vi "GEN_Time-coded_overlay_PIC.vi"(7 "Image size":cluster{"x":i32, "y":i32}={"x"=480, "y"=480}, 8 "Error In":errorcluster, 9 "Samples full merge, every N":i32=10000, 10 "Multiline grouping, samples":i32=100, 11 "Full track array":T1(array[cluster])) -> (0 "Error Out":errorcluster, 3 "Time-coded overlay pixmap":u32[][](array[numeric]) format="%x")   [LabVIEW 2018, in "Tracker.lvlib"]
uses:
  Tracker.lvlib
  Controls/CTL_Color_ramp.ctl
  Common_Resources.lvlib
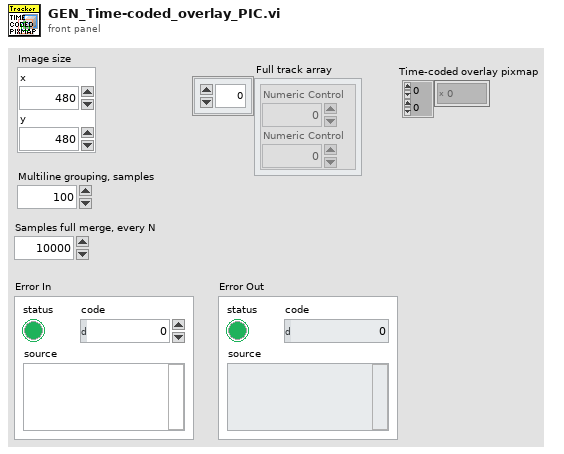
[diagram p1: front panel]
types:
  T1 = cluster{"Numeric Control":dbl, "Numeric Control":dbl}[]
  T2 = typedef "Common_Resources.lvlib/CTL_Color_ramp.ctl" = u32[]
  T3 = cluster{"Left":i32, "Top":i32, "Right":i32, "Bottom":i32}
  T4 = cluster{"Width":i16, "Style":enum32{"Solid", "Dash", "Dot", "DashDot", "DashDotDot"}}
  T5 = cluster{"Numeric Control":dbl, "Numeric Control":dbl}
  T6 = cluster{"Width":u16, "Style":enum32{"Solid", "Dash", "Dot", "DashDot", "DashDotDot"}}
  T7 = typedef "imagedata.ctl" = cluster{"image type":i32, "image depth":i32, "image":u8[], "mask":u8[], "colors":u32[], "Rectangle":cluster{"left":i16, "top":i16, "right":i16, "bottom":i16}}
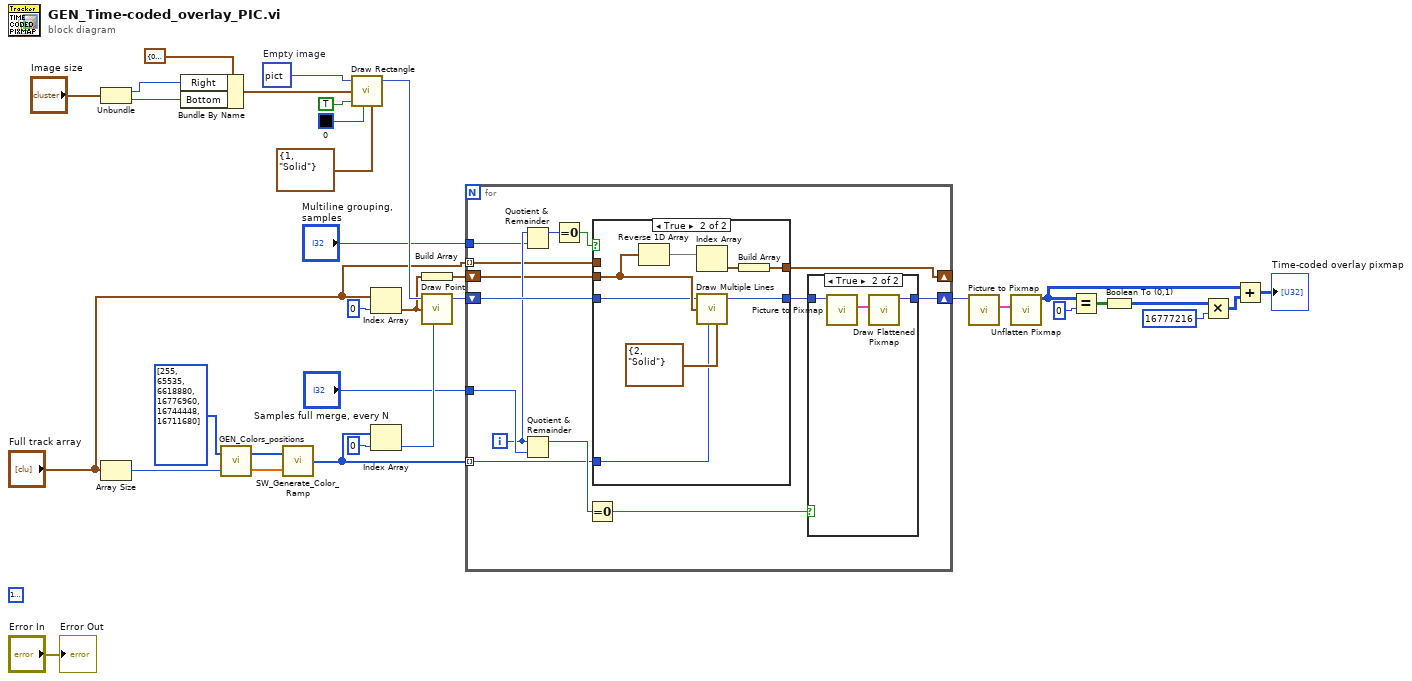
[diagram p0: block diagram]
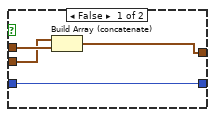
[diagram p2: hidden frame]
diagram:
  (unwired) u32 16777216
  w18 = picture data[5B]  # Empty image
  n1 = Unbundle("Image size") -> ("x"=w32:i32, "y"=w33:i32)
  n2 = Array Size(array="Full track array") -> (size(s)=w13:i32)
  n3 = Bundle By Name(cluster=T3 {"Left"=0, "Top"=0, "Right"=0, "Bottom"=0} ("Rectangle"), "Right"=w32, "Bottom"=w33) -> (w34:T3)
  n4 = call "GEN_Colors_positions.vi"("Highest color position"=w13, "Initial colors ramp array in"=T2 [255, 65535, 6618880, 16776960, 16744448, 16711680] ("Initial colors ramp array")) -> ("Colors positions"=w15:dbl[], "Initial colors ramp array out"=w16:T2)
  n5 = call "SW_Generate_Color_Ramp.vi"("Colors rel. pos."=w15, "Colors array"=w16) -> ("Colors array"=w11:u32[])
  n6 = call <vilib>:"Draw Rectangle.vi"("picture"=w18, "rect"=w34, "fill?(F)"=TRUE, "color(black)"=u32 0, "pen"=T4 {"Width"=1, "Style"=enum."Solid"}) -> ("new picture"=w28:picture)  [unwired: 4 in]
  n7 = Index Array(array="Full track array", index=0) -> (element=w23:T5)
  n8 = Index Array(array=w11, index=0) -> (element=w29:u32)
  n9 = Build Array(w23) -> (w24:T1)
  n10 = call <vilib>:"Draw Point.vi"("picture"=w28, "point(x,y)"=w23, "color(black)"=w29) -> ("new picture"=w22:picture)  [unwired: 6 in]
  n11 = for {
    shift-right: [w45] -> w25
    shift-left: w22 -> [w44]
    tunnel: "Full track array" -> [w39] mode=indexing
    tunnel: w11 -> [w36] mode=indexing
    tunnel: "Samples full merge, every N" -> [w46]
    tunnel: "Multiline grouping, samples" -> [w41]
    shift-right: [w37] -> _
    shift-left: w24 -> [w38]
    i -> [w42]
    n12 = Quotient & Remainder(x=w42, y=w41) -> (x-y*floor(x/y)=w43:i32)  [unwired: 1 out]
    n13 = Quotient & Remainder(x=w42, y=w46) -> (x-y*floor(x/y)=w47:i32)  [unwired: 1 out]
    n14 = Equal To 0?(x=w43) -> (x = 0?=w35:bool)
    n15 = Equal To 0?(x=w47) -> (x = 0?=w48:bool)
    n16 = case shown="True" w35 {
      tunnel: w44 -> [w52 w55]
      tunnel: [w52 w54] -> w40
      tunnel: w39 -> [w51 _]
      tunnel: w38 -> [w50 w56]
      tunnel: [w49 w53] -> w37
      tunnel: w36 -> [_ w57]
      frame False {
        n17 = Build Array (concatenate)(w50, w51) -> (w49:T1)
      }
      frame True {
        n18 = Reverse 1D Array(array=w56) -> (reversed array=w60:T1)
        n19 = Index Array(array=w60) -> (element=w59:T5)  [unwired: 1 in]
        n20 = call <vilib>:"Draw Multiple Lines.vi"("picture"=w55, "line endpoints"=w56, "color(black)"=w57, "pen"=T6 {"Width"=2, "Style"=enum."Solid"}) -> ("new picture"=w54:picture)  [unwired: 5 in]
        n21 = Build Array(w59) -> (w53:T1)
      }
    }
    n22 = case shown="True" w48 {
      tunnel: [w61 w63] -> w45
      tunnel: w40 -> [w61 w62]
      frame False {
      }
      frame True {
        n23 = call <vilib>:"Picture to Pixmap.vi"("picture"=w62) -> ("image data"=w64:T7)  [unwired: 9 in, 1 out]
        n24 = call <vilib>:"Draw Flattened Pixmap.vi"("image data"=w64) -> ("new picture"=w63:picture)  [unwired: 8 in]
      }
    }
  }
  n25 = call <vilib>:"Picture to Pixmap.vi"("picture"=w25) -> ("image data"=w10:T7)  [unwired: 9 in, 1 out]
  n26 = call <vilib>:"Unflatten Pixmap.vi"("image data"=w10) -> ("24-bit pixmap"=w2:u32[][])  [unwired: 4 in, 6 out]
  n27 = Equal?(x=w2, y=0) -> (x = y?=w6:bool[][])
  n28 = Boolean To (0,1)(Boolean=w6) -> (0, 1=w5:i16[][])
  n29 = Multiply(x=w5, y=16777216) -> (x*y=w3:i32[][])
  n30 = Add(x=w2, y=w3) -> (x+y=→"Time-coded overlay pixmap":u32[][])
  "Error Out" <- "Error In"
